vi "OutputSwerveDrive.vi"() -> ()   [LabVIEW 2020]
doc: "This VI runs feedback and feedforward controllers, manages safety interlocks, and sends commands to the swerve drive motors. This VI also controls the commanded drive shifter (low gear or high gear) state."
uses:
  <vilib>/Rock Robotics/WPI/Solenoid/WPI_SolenoidValue.ctl
  <vilib>/Rock Robotics/WPI/ThirdParty/Phoenix-LabVIEW/Motor Controller/Controls/CTRE_Phoenix_MotorControl_ControlMode.ctl
  <vilib>/Rock Robotics/WPI/ThirdParty/Phoenix-LabVIEW/Motor Controller/Controls/CTRE_Phoenix_MotorControl_NeutralMode.ctl
  21d1f6ed-8aa7-4c08-a7f4-4e12b9ae70b2.vi
  bd7bff45-d105-4c72-b52f-b7d898b15bf8.vi
  96bdb372-2377-4471-891f-ae36cd8cf6e7.vi
  4a6563c0-2600-4cc4-b814-5bfdd37bee33.vi
  59edaa1e-6d55-4e0d-9ccd-6771bdd34e38.vi
  9422521f-1ab3-4d1d-a0e1-edf0c1a6602b.vi
  164a13db-b17b-4981-8c2b-304dea5fbafc.vi
  bf4fe2dc-b12c-4808-b801-08a1d6a94233.vi
  9914bed3-0d1c-4b06-b050-22aab9a27a8c.vi
  dd2354c2-df0e-4340-ba82-09bb2e9cf5c3.vi
  13dda775-fe22-4909-989b-e16af49b0f34.vi
  2fe6b0e9-d121-4a66-8d55-455f8b7e1020.vi
  e77e916c-e179-4e89-92bf-a3cab155e43b.vi
  sensordata.vi
  refnumbers.vi
  GRNF_CTREMotor.vi
  <vilib>/Rock Robotics/WPI/ThirdParty/Phoenix-LabVIEW/Motor Controller/Get/CTRE_Phoenix_MotorController_GetSelectedSensorData.vi
  robotoutputs.vi
  driverdata.vi
  TAI_Motor.vi
  GRNF_GenericSolenoid.vi
  TAI_Solenoid.vi
  <vilib>/Rock Robotics/WPI/Solenoid/WPI_SolenoidSetEnum.vi
  autonomousinfo.vi
panel:
  in  "Force to Low Gear":bool
  in  "Force To High Gear":bool
  in  "Drive Command Override [0,1]":dbl min=0.0 max=1.0 step=0.1
  in  "Manually Override Drive Calibration":bool
  in  "Time Below Speed (ms)":u32=150
  in  "Time Above Speed (ms)":u32=150
  in  "Switch to Low Gear (rpm)":dbl=1000.0
  in  "Switch to High Gear (rpm)":dbl=3500.0
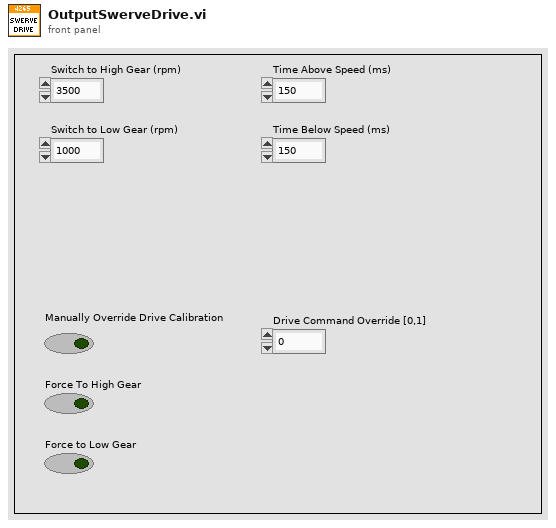
[diagram p1: front panel]
types:
  T1 = typedef "WPI_MotorControlDeviceRef.ctl" = cluster{"DeviceStatus":errorcluster, "Type":T2, "PWM":cluster{"PWM Channel":T3, "DeadBand":T4}, "CAN":cluster{"Device Number":u8, "SetOutput VI Ref":variant, "GetOutput VI Ref":variant, "Enable VI Ref":variant, "Disable VI Ref":variant, "Data":variant}, "Invert":bool, "DIO PWM":cluster{"PWM \"Enable\" Channel":T3, "DIOChannel":T5, "PWM Rate":dbl}}
  T2 = typedef "WPI_MotorControlType.ctl" = enum16{"PWM", "CAN", "DIO PWM"}
  T3 = typedef "FPGA_DIOPWMChannel.ctl" = enum8{"PWM 0", "PWM 1", "PWM 2", "PWM 3", "PWM 4", "PWM 5", "PWM 6", "PWM 7", "PWM 8", "PWM 9", "PWM MXP 0", "PWM MXP 1", "PWM MXP 2", "PWM MXP 3", "PWM MXP 4", "PWM MXP 5", "PWM MXP 6", "PWM MXP 7", "PWM MXP 8", "PWM MXP 9", "Invalid"}
  T4 = typedef "WPI_PWMDeadband.ctl" = cluster{"Name":string, "maxPositivePwm":i32, "minPositivePwm":i32, "centerPwm":i32, "maxNegativePwm":i32, "minNegativePwm":i32, "angularRange":u16}
  T5 = typedef "FPGA_DIOChannel.ctl" = enum8{"DIO 0", "DIO 1", "DIO 2", "DIO 3", "DIO 4", "DIO 5", "DIO 6", "DIO 7", "DIO 8", "DIO 9", "DIO MXP 0", "DIO MXP 1", "DIO MXP 2", "DIO MXP 3", "DIO MXP 4", "DIO MXP 5", "DIO MXP 6", "DIO MXP 7", "DIO MXP 8", "DIO MXP 9", "DIO MXP 10", "DIO MXP 11", "DIO MXP 12", "DIO MXP 13", "DIO MXP 14", "DIO MXP 15", "SPI Port CS1", "SPI Port CS2", "SPI Port CS3", "SPI Port MISO", "SPI Port MOSI", "Invalid"}
  T6 = enum16{"Low Gear", "High Gear", "Transiting", "Unknown", "Force Low Gear"}
  T7 = typedef "CTRE_Phoenix_MotorControl_NeutralMode.ctl" = enum8{"EEPROMSetting", "Override to Coast", "Override to Brake"}
  T8 = typedef "CTRE_Phoenix_MotorControl_ControlMode.ctl" = u16
  T9 = enum16{"No Changed Output", "New Normal Output", "New Testing Output"}
  T10 = typedef "WPI_SolenoidDevRef.ctl" = cluster{"DevStatus":errorcluster, "Pneumatics Control Module":u8, "Forward Solenoid Channel":T11, "Reverse Solenoid Channel":T11}
  T11 = typedef "WPI_SolenoidChannel.ctl" = enum8{"Solenoid 0", "Solenoid 1", "Solenoid 2", "Solenoid 3", "Solenoid 4", "Solenoid 5", "Solenoid 6", "Solenoid 7", "Solenoid 8", "Solenoid 9", "Solenoid 10", "Solenoid 11", "Solenoid 12", "Solenoid 13", "Solenoid 14", "Solenoid 15", "Invalid"}
  T12 = typedef "WPI_SolenoidValue.ctl" = enum16{"Off", "On", "Forward", "Reverse"}
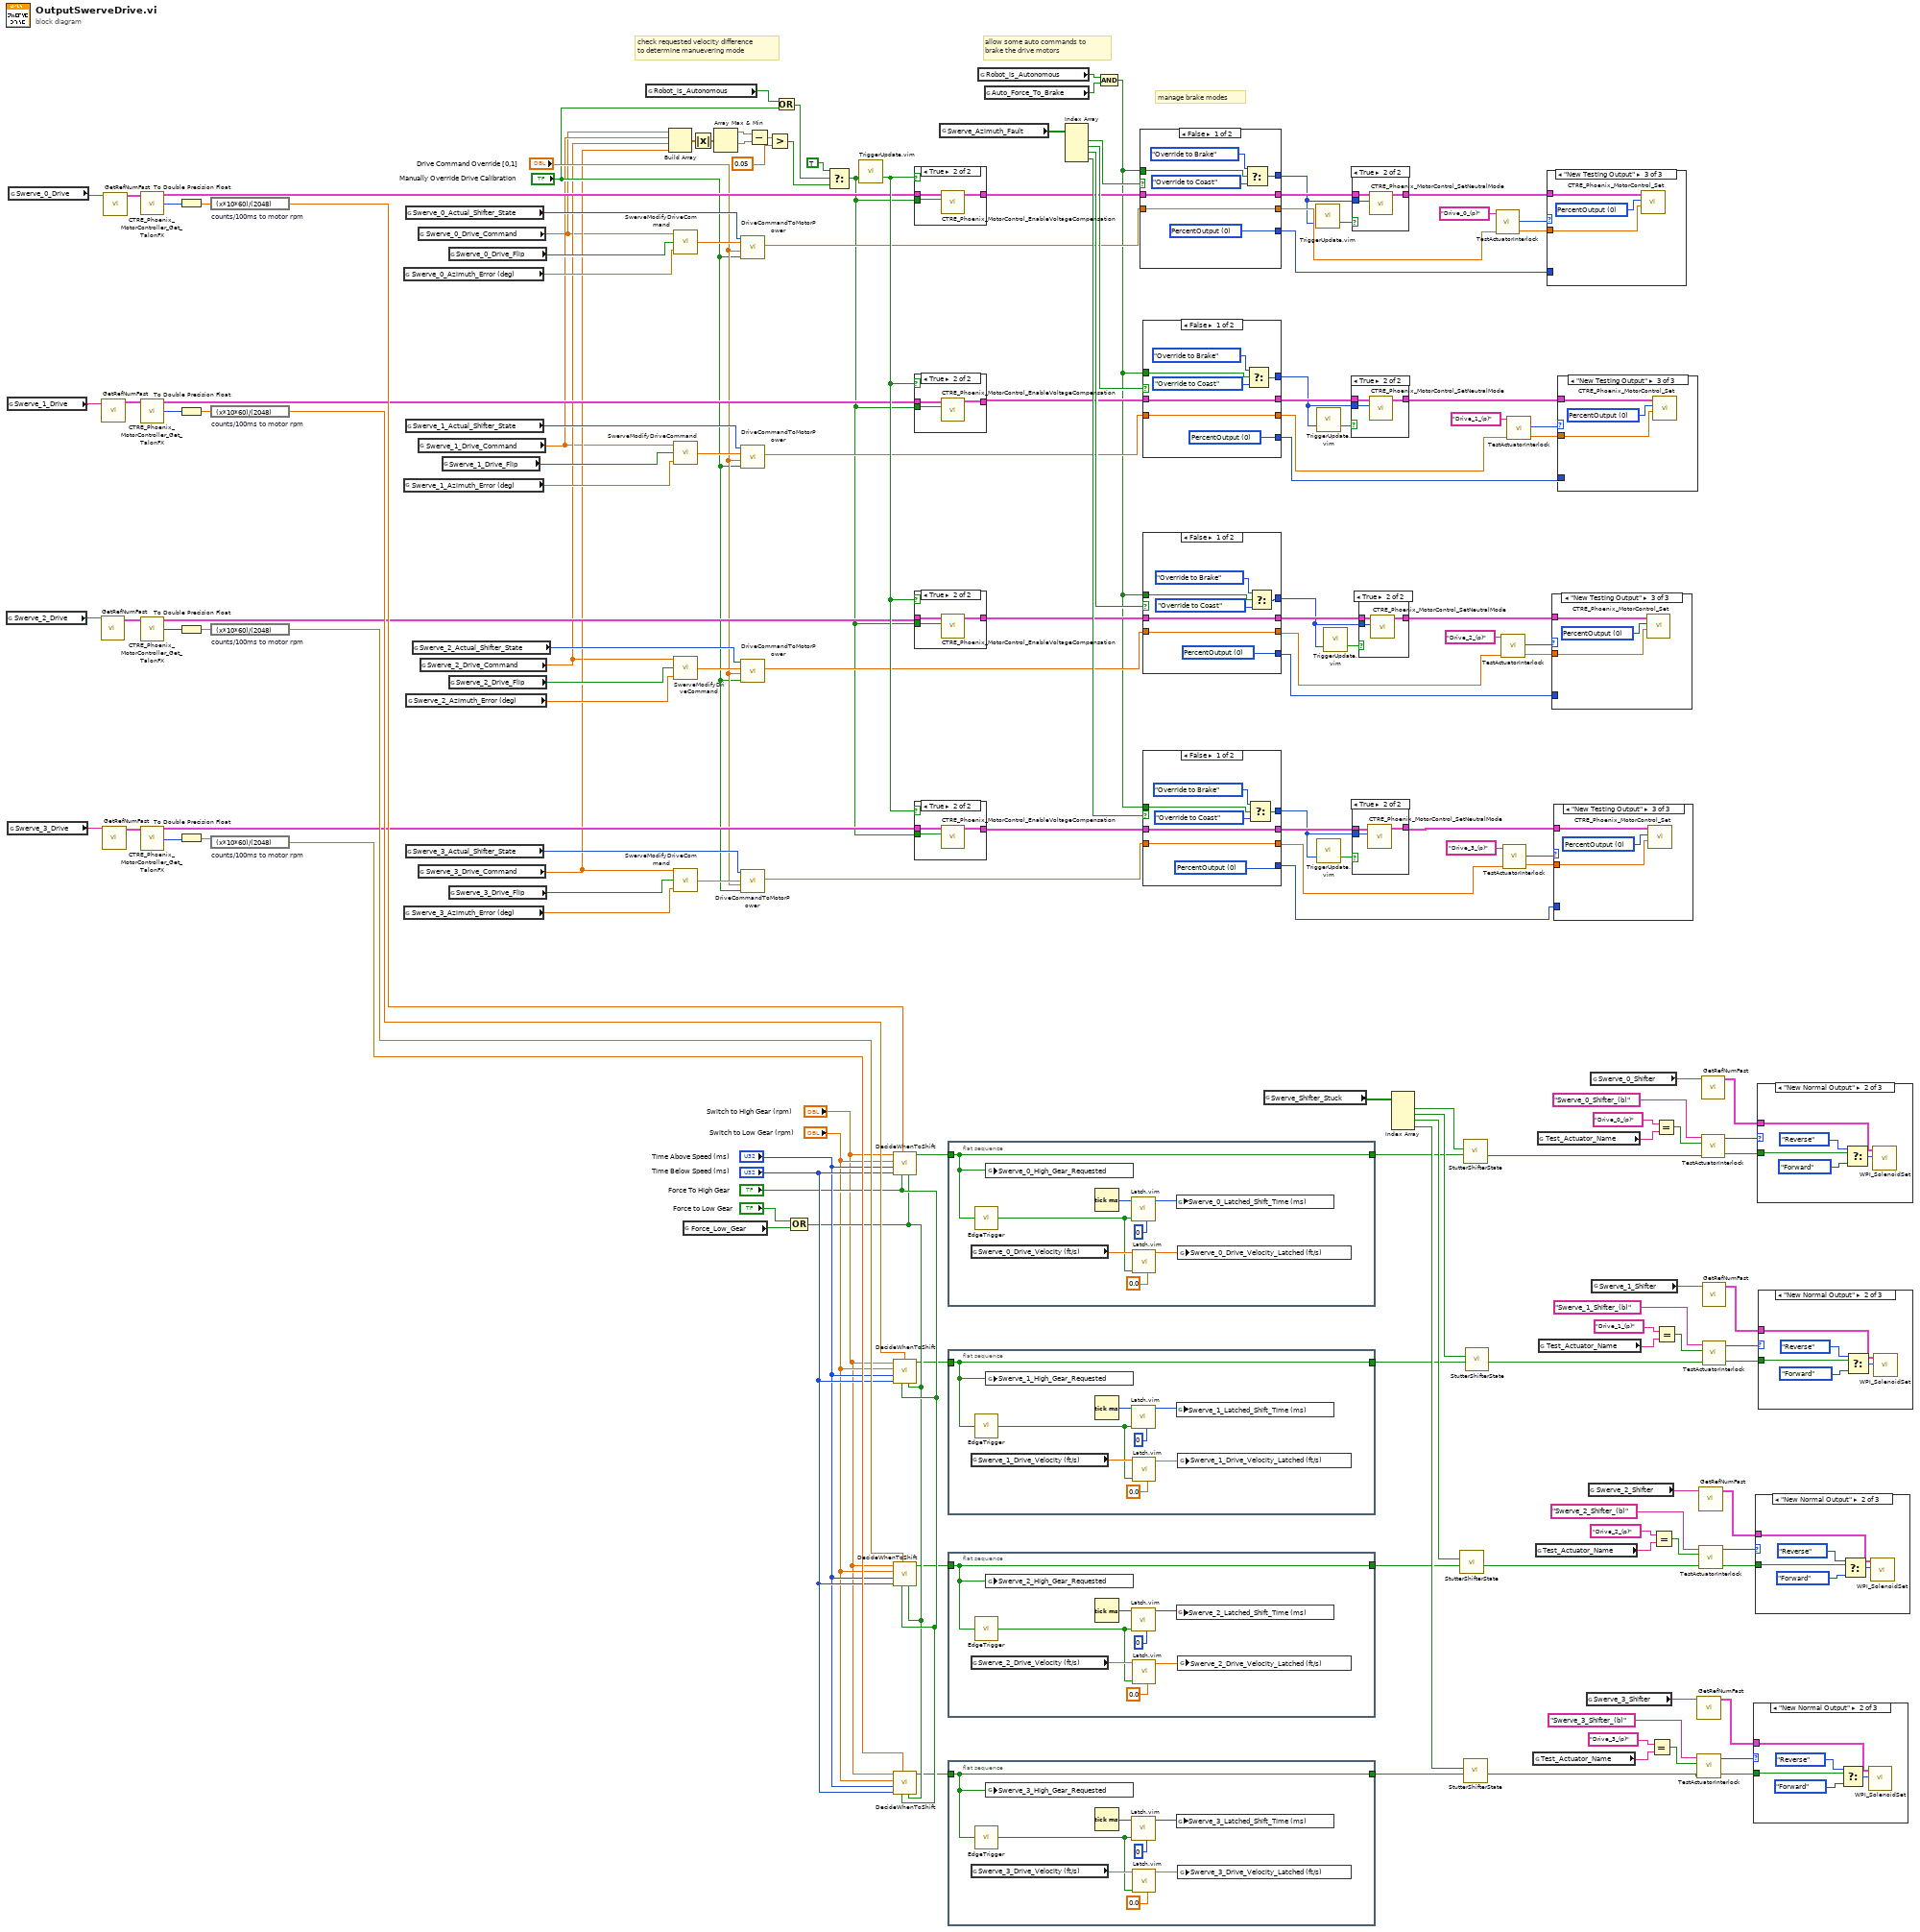
[diagram p0: block diagram]
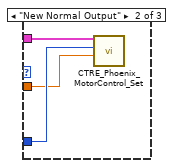
[diagram p3: hidden frame]
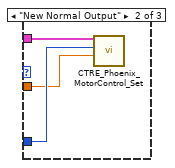
[diagram p5: hidden frame]
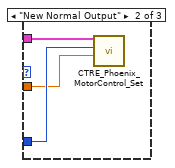
[diagram p7: hidden frame]
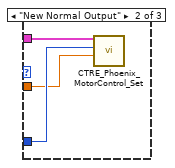
[diagram p9: hidden frame]
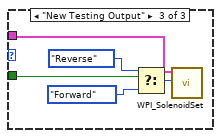
[diagram p11: hidden frame]
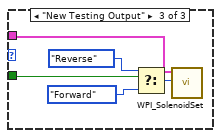
[diagram p13: hidden frame]
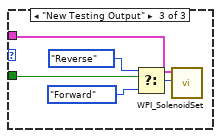
[diagram p15: hidden frame]
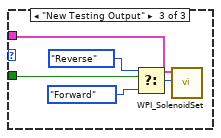
[diagram p17: hidden frame]
diagram:
  # "allow some auto commands to\nbrake the drive motors"
  # "check requested velocity difference\nto determine manuevering mode"
  # "manage brake modes"
  n1 = global read "refnumbers.vi" "Swerve_2_Drive"() -> (w164:string)
  n2 = global read "refnumbers.vi" "Swerve_1_Drive"() -> (w163:string)
  n3 = global read "refnumbers.vi" "Swerve_3_Drive"() -> (w165:string)
  n4 = global read "refnumbers.vi" "Swerve_0_Drive"() -> (w162:string)
  n5 = call-poly "GetRefNumFast.vi"("RefNum Name"=w164) -> ("Device Reference"=w131:T1)  [unwired: 5 in, 1 out]
  n6 = call-poly "GetRefNumFast.vi"("RefNum Name"=w163) -> ("Device Reference"=w132:T1)  [unwired: 5 in, 1 out]
  n7 = call-poly "GetRefNumFast.vi"("RefNum Name"=w165) -> ("Device Reference"=w130:T1)  [unwired: 5 in, 1 out]
  n8 = call-poly "GetRefNumFast.vi"("RefNum Name"=w162) -> ("Device Reference"=w133:T1)  [unwired: 5 in, 1 out]
  n9 = call-poly <vilib>:"CTRE_Phoenix_MotorController_Get_TalonFX.vi"("PhoenixMotorControlDevRef"=w133) -> ("PhoenixMotorControlDevRef"=w136:T1, "Velocity (Raw Sensor Units per 100 ms)"=w141:i32)  [unwired: 11 in, 2 out]
  n10 = call-poly <vilib>:"CTRE_Phoenix_MotorController_Get_TalonFX.vi"("PhoenixMotorControlDevRef"=w132) -> ("PhoenixMotorControlDevRef"=w134:T1, "Velocity (Raw Sensor Units per 100 ms)"=w140:i32)  [unwired: 11 in, 2 out]
  n11 = call-poly <vilib>:"CTRE_Phoenix_MotorController_Get_TalonFX.vi"("PhoenixMotorControlDevRef"=w131) -> ("PhoenixMotorControlDevRef"=w135:T1, "Velocity (Raw Sensor Units per 100 ms)"=w139:i32)  [unwired: 11 in, 2 out]
  n12 = call-poly <vilib>:"CTRE_Phoenix_MotorController_Get_TalonFX.vi"("PhoenixMotorControlDevRef"=w130) -> ("PhoenixMotorControlDevRef"=w125:T1, "Velocity (Raw Sensor Units per 100 ms)"=w138:i32)  [unwired: 11 in, 2 out]
  n13 = To Double Precision Float(number=w141) -> (double precision float=w148:dbl)
  n14 = To Double Precision Float(number=w140) -> (double precision float=w147:dbl)
  n15 = To Double Precision Float(number=w139) -> (double precision float=w146:dbl)
  n16 = To Double Precision Float(number=w138) -> (double precision float=w145:dbl)
  n17 = expression code="(x*10*60)/(2048)" "counts/100ms to motor rpm"(w148) -> (w142:dbl)
  n18 = expression code="(x*10*60)/(2048)" "counts/100ms to motor rpm"(w147) -> (w143:dbl)
  n19 = expression code="(x*10*60)/(2048)" "counts/100ms to motor rpm"(w146) -> (w144:dbl)
  n20 = expression code="(x*10*60)/(2048)" "counts/100ms to motor rpm"(w145) -> (w156:dbl)
  n21 = global read "robotoutputs.vi" "Swerve_0_Azimuth_Error (deg)"() -> (w101:dbl)
  n22 = global read "robotoutputs.vi" "Swerve_1_Azimuth_Error (deg)"() -> (w103:dbl)
  n23 = global read "robotoutputs.vi" "Swerve_3_Azimuth_Error (deg)"() -> (w137:dbl)
  n24 = global read "sensordata.vi" "Swerve_0_Actual_Shifter_State"() -> (w121:T6)
  n25 = global read "sensordata.vi" "Swerve_1_Actual_Shifter_State"() -> (w118:T6)
  n26 = global read "sensordata.vi" "Swerve_3_Actual_Shifter_State"() -> (w112:T6)
  n27 = global read "robotoutputs.vi" "Swerve_2_Azimuth_Error (deg)"() -> (w106:dbl)
  n28 = global read "sensordata.vi" "Swerve_2_Actual_Shifter_State"() -> (w116:T6)
  n29 = global read "robotoutputs.vi" "Swerve_0_Drive_Command"() -> (w5:dbl)
  n30 = global read "robotoutputs.vi" "Swerve_1_Drive_Command"() -> (w6:dbl)
  n31 = global read "robotoutputs.vi" "Swerve_3_Drive_Command"() -> (w8:dbl)
  n32 = global read "robotoutputs.vi" "Swerve_2_Drive_Command"() -> (w7:dbl)
  n33 = global read "robotoutputs.vi" "Swerve_1_Drive_Flip"() -> (w104:bool)
  n34 = global read "robotoutputs.vi" "Swerve_0_Drive_Flip"() -> (w100:bool)
  n35 = global read "robotoutputs.vi" "Swerve_2_Drive_Flip"() -> (w105:bool)
  n36 = global read "robotoutputs.vi" "Swerve_3_Drive_Flip"() -> (w102:bool)
  n37 = global read "driverdata.vi" "Robot_is_Autonomous"() -> (w108:bool)
  n38 = Build Array(w5, w6, w7, w8) -> (w155:dbl[])
  n39 = call "SwerveModifyDriveCommand.vi"("Azimuth Error (deg)"=w101, "Flip Drive Command"=w100, "Raw Drive Command (ul)"=w5) -> ("Modified Drive Command (ul)"=w122:dbl)
  n40 = call "SwerveModifyDriveCommand.vi"("Azimuth Error (deg)"=w103, "Flip Drive Command"=w104, "Raw Drive Command (ul)"=w6) -> ("Modified Drive Command (ul)"=w119:dbl)
  n41 = call "SwerveModifyDriveCommand.vi"("Azimuth Error (deg)"=w106, "Flip Drive Command"=w105, "Raw Drive Command (ul)"=w7) -> ("Modified Drive Command (ul)"=w115:dbl)
  n42 = call "SwerveModifyDriveCommand.vi"("Azimuth Error (deg)"=w137, "Flip Drive Command"=w102, "Raw Drive Command (ul)"=w8) -> ("Modified Drive Command (ul)"=w113:dbl)
  n43 = global read "robotoutputs.vi" "Force_Low_Gear"() -> (w89:bool)
  n44 = Absolute Value(x=w155) -> (abs(x)=w149:dbl[])
  n45 = Array Max & Min(array=w149) -> (max value=w154:dbl, min value=w153:dbl)  [unwired: 2 out]
  n46 = call "DriveCommandToMotorPower.vi"("Drive Command Override"="Manually Override Drive Calibration", "Drive Command Override (ul) [-1,1]"="Drive Command Override [0,1]", "Drive Command (ul) [-1,1]"=w122, "Actual Shifter State"=w121) -> ("Motor Power (ul) [-1,1]"=w120:dbl)  [unwired: 7 in]
  n47 = call "DriveCommandToMotorPower.vi"("Drive Command Override"="Manually Override Drive Calibration", "Drive Command Override (ul) [-1,1]"="Drive Command Override [0,1]", "Drive Command (ul) [-1,1]"=w119, "Actual Shifter State"=w118) -> ("Motor Power (ul) [-1,1]"=w117:dbl)  [unwired: 7 in]
  n48 = call "DriveCommandToMotorPower.vi"("Drive Command Override"="Manually Override Drive Calibration", "Drive Command Override (ul) [-1,1]"="Drive Command Override [0,1]", "Drive Command (ul) [-1,1]"=w115, "Actual Shifter State"=w116) -> ("Motor Power (ul) [-1,1]"=w114:dbl)  [unwired: 7 in]
  n49 = call "DriveCommandToMotorPower.vi"("Drive Command Override"="Manually Override Drive Calibration", "Drive Command Override (ul) [-1,1]"="Drive Command Override [0,1]", "Drive Command (ul) [-1,1]"=w113, "Actual Shifter State"=w112) -> ("Motor Power (ul) [-1,1]"=w111:dbl)  [unwired: 7 in]
  n50 = Subtract(x=w154, y=w153) -> (x-y=w152:dbl)
  n51 = Greater?(x=w152, y=0.05) -> (0:w123:bool)
  n52 = Or(x=w108, y="Manually Override Drive Calibration") -> (x .or. y?=w109:bool)
  n53 = Compound Arithmetic op=OR("Force to Low Gear", w89) -> (w90:bool)
  n54 = Select(t=TRUE, s=w109, f=w123) -> (s? t:f=w83:bool)
  n55 = call "TriggerUpdate.vim"("Trigger"=w83) -> ("Update"=w150:bool)  [unwired: 2 in]
  n56 = call "DecideWhenToShift.vi"("Force to Low Gear"=w90, "Force To High Gear"="Force To High Gear", "Drive Motor Speed (rpm)"=w142, "Time Below Speed (ms)"="Time Below Speed (ms)", "Time Above Speed (ms)"="Time Above Speed (ms)", "Switch to Low Gear (rpm)"="Switch to Low Gear (rpm)", "Switch to High Gear (rpm)"="Switch to High Gear (rpm)") -> ("Requested Shifter State"=w78:bool)  [unwired: 4 in]
  n57 = call "DecideWhenToShift.vi"("Force to Low Gear"=w90, "Force To High Gear"="Force To High Gear", "Drive Motor Speed (rpm)"=w143, "Time Below Speed (ms)"="Time Below Speed (ms)", "Time Above Speed (ms)"="Time Above Speed (ms)", "Switch to Low Gear (rpm)"="Switch to Low Gear (rpm)", "Switch to High Gear (rpm)"="Switch to High Gear (rpm)") -> ("Requested Shifter State"=w76:bool)  [unwired: 4 in]
  n58 = call "DecideWhenToShift.vi"("Force to Low Gear"=w90, "Force To High Gear"="Force To High Gear", "Drive Motor Speed (rpm)"=w144, "Time Below Speed (ms)"="Time Below Speed (ms)", "Time Above Speed (ms)"="Time Above Speed (ms)", "Switch to Low Gear (rpm)"="Switch to Low Gear (rpm)", "Switch to High Gear (rpm)"="Switch to High Gear (rpm)") -> ("Requested Shifter State"=w74:bool)  [unwired: 4 in]
  n59 = call "DecideWhenToShift.vi"("Force to Low Gear"=w90, "Force To High Gear"="Force To High Gear", "Drive Motor Speed (rpm)"=w156, "Time Below Speed (ms)"="Time Below Speed (ms)", "Time Above Speed (ms)"="Time Above Speed (ms)", "Switch to Low Gear (rpm)"="Switch to Low Gear (rpm)", "Switch to High Gear (rpm)"="Switch to High Gear (rpm)") -> ("Requested Shifter State"=w72:bool)  [unwired: 4 in]
  n60 = case shown="True" w150 {
    tunnel: w136 -> [w168 w171]
    tunnel: [w168 w170] -> w129
    tunnel: w83 -> [_ w169]
    frame False {
    }
    frame True {
      n61 = call <vilib>:"CTRE_Phoenix_MotorControl_EnableVoltageCompensation.vi"("Enable Voltage Compensation?"=w169, "PhoenixMotorControlDevRef"=w171) -> ("PhoenixMotorControlDevRef"=w170:T1)  [unwired: 8 in, 1 out]
    }
  }
  n62 = case shown="True" w150 {
    tunnel: w134 -> [w172 w175]
    tunnel: [w172 w174] -> w128
    tunnel: w83 -> [_ w173]
    frame False {
    }
    frame True {
      n63 = call <vilib>:"CTRE_Phoenix_MotorControl_EnableVoltageCompensation.vi"("Enable Voltage Compensation?"=w173, "PhoenixMotorControlDevRef"=w175) -> ("PhoenixMotorControlDevRef"=w174:T1)  [unwired: 8 in, 1 out]
    }
  }
  n64 = case shown="True" w150 {
    tunnel: w135 -> [w176 w179]
    tunnel: [w176 w178] -> w127
    tunnel: w83 -> [_ w177]
    frame False {
    }
    frame True {
      n65 = call <vilib>:"CTRE_Phoenix_MotorControl_EnableVoltageCompensation.vi"("Enable Voltage Compensation?"=w177, "PhoenixMotorControlDevRef"=w179) -> ("PhoenixMotorControlDevRef"=w178:T1)  [unwired: 8 in, 1 out]
    }
  }
  n66 = case shown="True" w150 {
    tunnel: [w180 w183] -> w126
    tunnel: w83 -> [_ w182]
    tunnel: w125 -> [w180 w181]
    frame False {
    }
    frame True {
      n67 = call <vilib>:"CTRE_Phoenix_MotorControl_EnableVoltageCompensation.vi"("Enable Voltage Compensation?"=w182, "PhoenixMotorControlDevRef"=w181) -> ("PhoenixMotorControlDevRef"=w183:T1)  [unwired: 8 in, 1 out]
    }
  }
  n68 = global read "sensordata.vi" "Swerve_Azimuth_Fault"() -> (w167:bool[])
  n69 = flat-sequence {
    tunnel: w78 -> [w191]
    tunnel: [w191] -> w77
    frame #0 {
      n70 = global read "sensordata.vi" "Swerve_0_Drive_Velocity (ft/s)"() -> (w188:dbl)
      n71 = call "EdgeTrigger.vi"("Input Signal"=w191) -> ("All Edge Trigger"=w186:bool)  [unwired: 2 out]
      n72 = global write "robotoutputs.vi" "Swerve_0_High_Gear_Requested"(w191) -> ()
      n73 = Tick Count (ms)() -> (millisecond timer value=w190:u32)
      n74 = call "Latch.vim"("Default Value"=u32 0 ("millisecond timer value"), "Latch Signal"=w186, "Latch Value"=w190) -> ("Latched"=w184:u32)  [unwired: 8 in]
      n75 = call "Latch.vim"("Default Value"=0.0, "Latch Signal"=w186, "Latch Value"=w188) -> ("Latched"=w185:dbl)  [unwired: 8 in]
      n76 = global write "sensordata.vi" "Swerve_0_Latched_Shift_Time (ms)"(w184) -> ()
      n77 = global write "sensordata.vi" "Swerve_0_Drive_Velocity_Latched (ft/s)"(w185) -> ()
    }
  }
  n78 = flat-sequence {
    tunnel: w76 -> [w199]
    tunnel: [w199] -> w75
    frame #0 {
      n79 = global read "sensordata.vi" "Swerve_1_Drive_Velocity (ft/s)"() -> (w196:dbl)
      n80 = call "EdgeTrigger.vi"("Input Signal"=w199) -> ("All Edge Trigger"=w194:bool)  [unwired: 2 out]
      n81 = global write "robotoutputs.vi" "Swerve_1_High_Gear_Requested"(w199) -> ()
      n82 = Tick Count (ms)() -> (millisecond timer value=w198:u32)
      n83 = call "Latch.vim"("Default Value"=u32 0 ("millisecond timer value"), "Latch Signal"=w194, "Latch Value"=w198) -> ("Latched"=w192:u32)  [unwired: 8 in]
      n84 = call "Latch.vim"("Default Value"=0.0, "Latch Signal"=w194, "Latch Value"=w196) -> ("Latched"=w193:dbl)  [unwired: 8 in]
      n85 = global write "sensordata.vi" "Swerve_1_Latched_Shift_Time (ms)"(w192) -> ()
      n86 = global write "sensordata.vi" "Swerve_1_Drive_Velocity_Latched (ft/s)"(w193) -> ()
    }
  }
  n87 = flat-sequence {
    tunnel: w74 -> [w207]
    tunnel: [w207] -> w73
    frame #0 {
      n88 = global read "sensordata.vi" "Swerve_2_Drive_Velocity (ft/s)"() -> (w204:dbl)
      n89 = call "EdgeTrigger.vi"("Input Signal"=w207) -> ("All Edge Trigger"=w202:bool)  [unwired: 2 out]
      n90 = global write "robotoutputs.vi" "Swerve_2_High_Gear_Requested"(w207) -> ()
      n91 = Tick Count (ms)() -> (millisecond timer value=w206:u32)
      n92 = call "Latch.vim"("Default Value"=u32 0 ("millisecond timer value"), "Latch Signal"=w202, "Latch Value"=w206) -> ("Latched"=w200:u32)  [unwired: 8 in]
      n93 = call "Latch.vim"("Default Value"=0.0, "Latch Signal"=w202, "Latch Value"=w204) -> ("Latched"=w201:dbl)  [unwired: 8 in]
      n94 = global write "sensordata.vi" "Swerve_2_Latched_Shift_Time (ms)"(w200) -> ()
      n95 = global write "sensordata.vi" "Swerve_2_Drive_Velocity_Latched (ft/s)"(w201) -> ()
    }
  }
  n96 = flat-sequence {
    tunnel: w72 -> [w215]
    tunnel: [w215] -> w71
    frame #0 {
      n97 = global read "sensordata.vi" "Swerve_3_Drive_Velocity (ft/s)"() -> (w212:dbl)
      n98 = call "EdgeTrigger.vi"("Input Signal"=w215) -> ("All Edge Trigger"=w210:bool)  [unwired: 2 out]
      n99 = global write "robotoutputs.vi" "Swerve_3_High_Gear_Requested"(w215) -> ()
      n100 = Tick Count (ms)() -> (millisecond timer value=w214:u32)
      n101 = call "Latch.vim"("Default Value"=u32 0 ("millisecond timer value"), "Latch Signal"=w210, "Latch Value"=w214) -> ("Latched"=w208:u32)  [unwired: 8 in]
      n102 = call "Latch.vim"("Default Value"=0.0, "Latch Signal"=w210, "Latch Value"=w212) -> ("Latched"=w209:dbl)  [unwired: 8 in]
      n103 = global write "sensordata.vi" "Swerve_3_Latched_Shift_Time (ms)"(w208) -> ()
      n104 = global write "sensordata.vi" "Swerve_3_Drive_Velocity_Latched (ft/s)"(w209) -> ()
    }
  }
  n105 = global read "driverdata.vi" "Robot_is_Autonomous"() -> (w3:bool)
  n106 = global read "autonomousinfo.vi" "Auto_Force_To_Brake"() -> (w2:bool)
  n107 = Index Array(array=w167) -> (element #1=w159:bool, element #2=w158:bool, element #3=w157:bool, element #4=w166:bool)  [unwired: 4 in]
  n108 = And(x=w3, y=w2) -> (x .and. y?=w1:bool)
  n109 = case shown="False" w159 {
    tunnel: [w222 w226] -> w82
    tunnel: w129 -> [w222 w226]
    tunnel: [w221 0.0 ("Command")] -> w160
    tunnel: w120 -> [w221 _]
    tunnel: [w220 w224] -> w33
    tunnel: [w219 CTRE_Phoenix_MotorControl_NeutralMode."Override to Coast" ("Motor Control Neutral Mode")] -> w70
    tunnel: w1 -> [w216 _]
    frame False {
      w220 = T8 0 items=["PercentOutput"=0, "Position"=1, "Velocity"=2, "Current"=3, "Follower"=5, "MotionProfile"=6, "MotionMagic"=7, "MotionProfileArc"=10, "Disabled"=15] ("Control Mode")
      n110 = Select(t=CTRE_Phoenix_MotorControl_NeutralMode."Override to Brake" ("Motor Control Neutral Mode"), s=w216, f=CTRE_Phoenix_MotorControl_NeutralMode."Override to Coast") -> (s? t:f=w219:T7)
    }
    frame True {
      w224 = T8 0 items=["PercentOutput"=0, "Position"=1, "Velocity"=2, "Current"=3, "Follower"=5, "MotionProfile"=6, "MotionMagic"=7, "MotionProfileArc"=10, "Disabled"=15] ("Control Mode")
    }
  }
  n111 = case shown="False" w158 {
    tunnel: [w233 w237] -> w81
    tunnel: w128 -> [w233 w237]
    tunnel: [w232 0.0 ("Command")] -> w27
    tunnel: w117 -> [w232 _]
    tunnel: [w231 w235] -> w26
    tunnel: [w228 CTRE_Phoenix_MotorControl_NeutralMode."Override to Coast" ("Motor Control Neutral Mode")] -> w68
    tunnel: w1 -> [w227 _]
    frame False {
      w231 = T8 0 items=["PercentOutput"=0, "Position"=1, "Velocity"=2, "Current"=3, "Follower"=5, "MotionProfile"=6, "MotionMagic"=7, "MotionProfileArc"=10, "Disabled"=15] ("Control Mode")
      n112 = Select(t=CTRE_Phoenix_MotorControl_NeutralMode."Override to Brake" ("Motor Control Neutral Mode"), s=w227, f=CTRE_Phoenix_MotorControl_NeutralMode."Override to Coast") -> (s? t:f=w228:T7)
    }
    frame True {
      w235 = T8 0 items=["PercentOutput"=0, "Position"=1, "Velocity"=2, "Current"=3, "Follower"=5, "MotionProfile"=6, "MotionMagic"=7, "MotionProfileArc"=10, "Disabled"=15] ("Control Mode")
    }
  }
  n113 = case shown="False" w157 {
    tunnel: [w244 w248] -> w80
    tunnel: w127 -> [w244 w248]
    tunnel: [w243 0.0 ("Command")] -> w20
    tunnel: w114 -> [w243 _]
    tunnel: [w242 w246] -> w19
    tunnel: [w239 CTRE_Phoenix_MotorControl_NeutralMode."Override to Coast" ("Motor Control Neutral Mode")] -> w65
    tunnel: w1 -> [w238 _]
    frame False {
      w242 = T8 0 items=["PercentOutput"=0, "Position"=1, "Velocity"=2, "Current"=3, "Follower"=5, "MotionProfile"=6, "MotionMagic"=7, "MotionProfileArc"=10, "Disabled"=15] ("Control Mode")
      n114 = Select(t=CTRE_Phoenix_MotorControl_NeutralMode."Override to Brake" ("Motor Control Neutral Mode"), s=w238, f=CTRE_Phoenix_MotorControl_NeutralMode."Override to Coast") -> (s? t:f=w239:T7)
    }
    frame True {
      w246 = T8 0 items=["PercentOutput"=0, "Position"=1, "Velocity"=2, "Current"=3, "Follower"=5, "MotionProfile"=6, "MotionMagic"=7, "MotionProfileArc"=10, "Disabled"=15] ("Control Mode")
    }
  }
  n115 = case shown="False" w166 {
    tunnel: [w255 w259] -> w79
    tunnel: w126 -> [w255 w259]
    tunnel: [w254 0.0 ("Command")] -> w14
    tunnel: w111 -> [w254 _]
    tunnel: [w253 w257] -> w13
    tunnel: [w250 CTRE_Phoenix_MotorControl_NeutralMode."Override to Coast" ("Motor Control Neutral Mode")] -> w63
    tunnel: w1 -> [w249 _]
    frame False {
      w253 = T8 0 items=["PercentOutput"=0, "Position"=1, "Velocity"=2, "Current"=3, "Follower"=5, "MotionProfile"=6, "MotionMagic"=7, "MotionProfileArc"=10, "Disabled"=15] ("Control Mode")
      n116 = Select(t=CTRE_Phoenix_MotorControl_NeutralMode."Override to Brake" ("Motor Control Neutral Mode"), s=w249, f=CTRE_Phoenix_MotorControl_NeutralMode."Override to Coast") -> (s? t:f=w250:T7)
    }
    frame True {
      w257 = T8 0 items=["PercentOutput"=0, "Position"=1, "Velocity"=2, "Current"=3, "Follower"=5, "MotionProfile"=6, "MotionMagic"=7, "MotionProfileArc"=10, "Disabled"=15] ("Control Mode")
    }
  }
  n117 = global read "sensordata.vi" "Swerve_Shifter_Stuck"() -> (w88:bool[])
  n118 = call "TriggerUpdate.vim"("Trigger"=w70) -> ("Update"=w69:bool)  [unwired: 2 in]
  n119 = call "TriggerUpdate.vim"("Trigger"=w68) -> ("Update"=w67:bool)  [unwired: 2 in]
  n120 = call "TriggerUpdate.vim"("Trigger"=w63) -> ("Update"=w64:bool)  [unwired: 2 in]
  n121 = call "TriggerUpdate.vim"("Trigger"=w65) -> ("Update"=w66:bool)  [unwired: 2 in]
  n122 = case shown="True" w67 {
    tunnel: w81 -> [w260 w263]
    tunnel: [w260 w262] -> w25
    tunnel: w68 -> [_ w261]
    frame False {
    }
    frame True {
      n123 = call <vilib>:"CTRE_Phoenix_MotorControl_SetNeutralMode.vi"("Motor Control Neutral Mode"=w261, "PhoenixMotorControlDevRef"=w263) -> ("PhoenixMotorControlDevRef"=w262:T1)  [unwired: 8 in, 1 out]
    }
  }
  n124 = case shown="True" w69 {
    tunnel: w70 -> [_ w267]
    tunnel: w82 -> [w264 w266]
    tunnel: [w264 w265] -> w31
    frame False {
    }
    frame True {
      n125 = call <vilib>:"CTRE_Phoenix_MotorControl_SetNeutralMode.vi"("Motor Control Neutral Mode"=w267, "PhoenixMotorControlDevRef"=w266) -> ("PhoenixMotorControlDevRef"=w265:T1)  [unwired: 8 in, 1 out]
    }
  }
  n126 = case shown="True" w64 {
    tunnel: w79 -> [w268 w271]
    tunnel: [w268 w270] -> w15
    tunnel: w63 -> [_ w269]
    frame False {
    }
    frame True {
      n127 = call <vilib>:"CTRE_Phoenix_MotorControl_SetNeutralMode.vi"("Motor Control Neutral Mode"=w269, "PhoenixMotorControlDevRef"=w271) -> ("PhoenixMotorControlDevRef"=w270:T1)  [unwired: 8 in, 1 out]
    }
  }
  n128 = case shown="True" w66 {
    tunnel: w80 -> [w272 w275]
    tunnel: [w272 w274] -> w21
    tunnel: w65 -> [_ w273]
    frame False {
    }
    frame True {
      n129 = call <vilib>:"CTRE_Phoenix_MotorControl_SetNeutralMode.vi"("Motor Control Neutral Mode"=w273, "PhoenixMotorControlDevRef"=w275) -> ("PhoenixMotorControlDevRef"=w274:T1)  [unwired: 8 in, 1 out]
    }
  }
  n130 = Index Array(array=w88) -> (element #1=w87:bool, element #2=w86:bool, element #3=w85:bool, element #4=w84:bool)  [unwired: 4 in]
  n131 = call "StutterShifterState.vi"("Requested Shifter State"=w73, "Request Stutter"=w85) -> ("Stuttered Shifter State"=w10:bool)  [unwired: 9 in]
  n132 = call "StutterShifterState.vi"("Requested Shifter State"=w77, "Request Stutter"=w87) -> ("Stuttered Shifter State"=w12:bool)  [unwired: 9 in]
  n133 = call "StutterShifterState.vi"("Requested Shifter State"=w71, "Request Stutter"=w84) -> ("Stuttered Shifter State"=w9:bool)  [unwired: 9 in]
  n134 = call "StutterShifterState.vi"("Requested Shifter State"=w75, "Request Stutter"=w86) -> ("Stuttered Shifter State"=w11:bool)  [unwired: 9 in]
  n135 = call-poly "TestActuatorInterlock.vi"("Normal Output"=w160, "Actuator Name"="Drive_0_(p)" ("Actuator_Name")) -> ("Interlocked Output"=w32:dbl, "Output Mode"=w34:T9)  [unwired: 3 in]
  n136 = call-poly "TestActuatorInterlock.vi"("Normal Output"=w20, "Actuator Name"="Drive_2_(p)" ("Actuator_Name")) -> ("Interlocked Output"=w22:dbl, "Output Mode"=w23:T9)  [unwired: 3 in]
  n137 = call-poly "TestActuatorInterlock.vi"("Normal Output"=w14, "Actuator Name"="Drive_3_(p)" ("Actuator_Name")) -> ("Interlocked Output"=w16:dbl, "Output Mode"=w17:T9)  [unwired: 3 in]
  n138 = call-poly "TestActuatorInterlock.vi"("Normal Output"=w27, "Actuator Name"="Drive_1_(p)" ("Actuator_Name")) -> ("Interlocked Output"=w28:dbl, "Output Mode"=w29:T9)  [unwired: 3 in]
  n139 = global read "driverdata.vi" "Test_Actuator_Name"() -> (w96:string)
  n140 = global read "driverdata.vi" "Test_Actuator_Name"() -> (w55:string)
  n141 = global read "driverdata.vi" "Test_Actuator_Name"() -> (w39:string)
  n142 = global read "driverdata.vi" "Test_Actuator_Name"() -> (w47:string)
  n143 = case shown="\"New Testing Output\"" w34 {
    tunnel: w33 -> [_ w278 _]
    tunnel: w31 -> [_ w276 w280]
    tunnel: w32 -> [_ w277 w279]
    frame "No Changed Output", Default {
    }
    frame "New Normal Output" {
      n144 = call <vilib>:"CTRE_Phoenix_MotorControl_Set.vi"("Output"=w277, "Control Mode"=w278, "PhoenixMotorControlDevRef"=w276) -> ()  [unwired: 7 in, 2 out]
    }
    frame "New Testing Output" {
      w281 = T8 0 items=["PercentOutput"=0, "Position"=1, "Velocity"=2, "Current"=3, "Follower"=5, "MotionProfile"=6, "MotionMagic"=7, "MotionProfileArc"=10, "Disabled"=15] ("Control Mode")
      n145 = call <vilib>:"CTRE_Phoenix_MotorControl_Set.vi"("Output"=w279, "Control Mode"=w281, "PhoenixMotorControlDevRef"=w280) -> ()  [unwired: 7 in, 2 out]
    }
  }
  n146 = case shown="\"New Testing Output\"" w23 {
    tunnel: w19 -> [_ w284 _]
    tunnel: w21 -> [_ w282 w286]
    tunnel: w22 -> [_ w283 w285]
    frame "No Changed Output", Default {
    }
    frame "New Normal Output" {
      n147 = call <vilib>:"CTRE_Phoenix_MotorControl_Set.vi"("Output"=w283, "Control Mode"=w284, "PhoenixMotorControlDevRef"=w282) -> ()  [unwired: 7 in, 2 out]
    }
    frame "New Testing Output" {
      w287 = T8 0 items=["PercentOutput"=0, "Position"=1, "Velocity"=2, "Current"=3, "Follower"=5, "MotionProfile"=6, "MotionMagic"=7, "MotionProfileArc"=10, "Disabled"=15] ("Control Mode")
      n148 = call <vilib>:"CTRE_Phoenix_MotorControl_Set.vi"("Output"=w285, "Control Mode"=w287, "PhoenixMotorControlDevRef"=w286) -> ()  [unwired: 7 in, 2 out]
    }
  }
  n149 = case shown="\"New Testing Output\"" w17 {
    tunnel: w13 -> [_ w290 _]
    tunnel: w15 -> [_ w288 w292]
    tunnel: w16 -> [_ w289 w291]
    frame "No Changed Output", Default {
    }
    frame "New Normal Output" {
      n150 = call <vilib>:"CTRE_Phoenix_MotorControl_Set.vi"("Output"=w289, "Control Mode"=w290, "PhoenixMotorControlDevRef"=w288) -> ()  [unwired: 7 in, 2 out]
    }
    frame "New Testing Output" {
      w293 = T8 0 items=["PercentOutput"=0, "Position"=1, "Velocity"=2, "Current"=3, "Follower"=5, "MotionProfile"=6, "MotionMagic"=7, "MotionProfileArc"=10, "Disabled"=15] ("Control Mode")
      n151 = call <vilib>:"CTRE_Phoenix_MotorControl_Set.vi"("Output"=w291, "Control Mode"=w293, "PhoenixMotorControlDevRef"=w292) -> ()  [unwired: 7 in, 2 out]
    }
  }
  n152 = case shown="\"New Testing Output\"" w29 {
    tunnel: w26 -> [_ w296 _]
    tunnel: w25 -> [_ w294 w298]
    tunnel: w28 -> [_ w295 w297]
    frame "No Changed Output", Default {
    }
    frame "New Normal Output" {
      n153 = call <vilib>:"CTRE_Phoenix_MotorControl_Set.vi"("Output"=w295, "Control Mode"=w296, "PhoenixMotorControlDevRef"=w294) -> ()  [unwired: 7 in, 2 out]
    }
    frame "New Testing Output" {
      w299 = T8 0 items=["PercentOutput"=0, "Position"=1, "Velocity"=2, "Current"=3, "Follower"=5, "MotionProfile"=6, "MotionMagic"=7, "MotionProfileArc"=10, "Disabled"=15] ("Control Mode")
      n154 = call <vilib>:"CTRE_Phoenix_MotorControl_Set.vi"("Output"=w297, "Control Mode"=w299, "PhoenixMotorControlDevRef"=w298) -> ()  [unwired: 7 in, 2 out]
    }
  }
  n155 = global read "refnumbers.vi" "Swerve_3_Shifter"() -> (w98:string)
  n156 = global read "refnumbers.vi" "Swerve_2_Shifter"() -> (w57:string)
  n157 = global read "refnumbers.vi" "Swerve_0_Shifter"() -> (w41:string)
  n158 = global read "refnumbers.vi" "Swerve_1_Shifter"() -> (w49:string)
  n159 = Equal?(x="Drive_3_(p)" ("Actuator_Name"), y=w96) -> (x = y?=w95:bool)
  n160 = Equal?(x="Drive_2_(p)" ("Actuator_Name"), y=w55) -> (x = y?=w54:bool)
  n161 = Equal?(x="Drive_0_(p)" ("Actuator_Name"), y=w39) -> (x = y?=w38:bool)
  n162 = Equal?(x="Drive_1_(p)" ("Actuator_Name"), y=w47) -> (x = y?=w46:bool)
  n163 = call-poly "GetRefNumFast.vi"("RefNum Name"=w98) -> ("Device Reference"=w59:T10)  [unwired: 5 in, 1 out]
  n164 = call-poly "TestActuatorInterlock.vi"("Normal Output"=w9, "Override Actuator Bypass"=w95, "Actuator Name"="Swerve_3_Shifter_(b)" ("Actuator_Name")) -> ("Interlocked Output"=w60:bool, "Output Mode"=w61:T9)  [unwired: 2 in]
  n165 = call-poly "GetRefNumFast.vi"("RefNum Name"=w57) -> ("Device Reference"=w51:T10)  [unwired: 5 in, 1 out]
  n166 = call-poly "TestActuatorInterlock.vi"("Normal Output"=w10, "Override Actuator Bypass"=w54, "Actuator Name"="Swerve_2_Shifter_(b)" ("Actuator_Name")) -> ("Interlocked Output"=w52:bool, "Output Mode"=w53:T9)  [unwired: 2 in]
  n167 = call-poly "GetRefNumFast.vi"("RefNum Name"=w41) -> ("Device Reference"=w35:T10)  [unwired: 5 in, 1 out]
  n168 = call-poly "TestActuatorInterlock.vi"("Normal Output"=w12, "Override Actuator Bypass"=w38, "Actuator Name"="Swerve_0_Shifter_(b)" ("Actuator_Name")) -> ("Interlocked Output"=w36:bool, "Output Mode"=w37:T9)  [unwired: 2 in]
  n169 = call-poly "GetRefNumFast.vi"("RefNum Name"=w49) -> ("Device Reference"=w43:T10)  [unwired: 5 in, 1 out]
  n170 = call-poly "TestActuatorInterlock.vi"("Normal Output"=w11, "Override Actuator Bypass"=w46, "Actuator Name"="Swerve_1_Shifter_(b)" ("Actuator_Name")) -> ("Interlocked Output"=w44:bool, "Output Mode"=w45:T9)  [unwired: 2 in]
  n171 = case shown="\"New Normal Output\"" w61 {
    tunnel: w60 -> [_ w301 w306]
    tunnel: w59 -> [_ w300 w305]
    frame "No Changed Output", Default {
    }
    frame "New Normal Output" {
      n172 = Select(t=WPI_SolenoidValue."Reverse" ("Value"), s=w301, f=WPI_SolenoidValue."Forward" ("Value")) -> (s? t:f=w302:T12)
      n173 = call-poly <vilib>:"WPI_SolenoidSet.vi"("Value"=w302, "SolenoidDevRef"=w300) -> ()  [unwired: 8 in, 2 out]
    }
    frame "New Testing Output" {
      n174 = Select(t=WPI_SolenoidValue."Reverse" ("Value"), s=w306, f=WPI_SolenoidValue."Forward" ("Value")) -> (s? t:f=w309:T12)
      n175 = call-poly <vilib>:"WPI_SolenoidSet.vi"("Value"=w309, "SolenoidDevRef"=w305) -> ()  [unwired: 8 in, 2 out]
    }
  }
  n176 = case shown="\"New Normal Output\"" w53 {
    tunnel: w52 -> [_ w311 w316]
    tunnel: w51 -> [_ w310 w315]
    frame "No Changed Output", Default {
    }
    frame "New Normal Output" {
      n177 = Select(t=WPI_SolenoidValue."Reverse" ("Value"), s=w311, f=WPI_SolenoidValue."Forward" ("Value")) -> (s? t:f=w312:T12)
      n178 = call-poly <vilib>:"WPI_SolenoidSet.vi"("Value"=w312, "SolenoidDevRef"=w310) -> ()  [unwired: 8 in, 2 out]
    }
    frame "New Testing Output" {
      n179 = Select(t=WPI_SolenoidValue."Reverse" ("Value"), s=w316, f=WPI_SolenoidValue."Forward" ("Value")) -> (s? t:f=w319:T12)
      n180 = call-poly <vilib>:"WPI_SolenoidSet.vi"("Value"=w319, "SolenoidDevRef"=w315) -> ()  [unwired: 8 in, 2 out]
    }
  }
  n181 = case shown="\"New Normal Output\"" w37 {
    tunnel: w36 -> [_ w321 w326]
    tunnel: w35 -> [_ w320 w325]
    frame "No Changed Output", Default {
    }
    frame "New Normal Output" {
      n182 = Select(t=WPI_SolenoidValue."Reverse" ("Value"), s=w321, f=WPI_SolenoidValue."Forward" ("Value")) -> (s? t:f=w322:T12)
      n183 = call-poly <vilib>:"WPI_SolenoidSet.vi"("Value"=w322, "SolenoidDevRef"=w320) -> ()  [unwired: 8 in, 2 out]
    }
    frame "New Testing Output" {
      n184 = Select(t=WPI_SolenoidValue."Reverse" ("Value"), s=w326, f=WPI_SolenoidValue."Forward" ("Value")) -> (s? t:f=w329:T12)
      n185 = call-poly <vilib>:"WPI_SolenoidSet.vi"("Value"=w329, "SolenoidDevRef"=w325) -> ()  [unwired: 8 in, 2 out]
    }
  }
  n186 = case shown="\"New Normal Output\"" w45 {
    tunnel: w44 -> [_ w331 w336]
    tunnel: w43 -> [_ w330 w335]
    frame "No Changed Output", Default {
    }
    frame "New Normal Output" {
      n187 = Select(t=WPI_SolenoidValue."Reverse" ("Value"), s=w331, f=WPI_SolenoidValue."Forward" ("Value")) -> (s? t:f=w332:T12)
      n188 = call-poly <vilib>:"WPI_SolenoidSet.vi"("Value"=w332, "SolenoidDevRef"=w330) -> ()  [unwired: 8 in, 2 out]
    }
    frame "New Testing Output" {
      n189 = Select(t=WPI_SolenoidValue."Reverse" ("Value"), s=w336, f=WPI_SolenoidValue."Forward" ("Value")) -> (s? t:f=w339:T12)
      n190 = call-poly <vilib>:"WPI_SolenoidSet.vi"("Value"=w339, "SolenoidDevRef"=w335) -> ()  [unwired: 8 in, 2 out]
    }
  }
